vi "END SEM PROJECT ECG AND TEMP.vi"() -> ()   [LabVIEW 2014]
uses:
  <vilib>/MakerHub/LINX/Public/Peripherals/Analog/Analog Read 1 Chan.vi
  <vilib>/MakerHub/LINX/Public/Peripherals/Digital/Digital Write 1 Chan.vi
  <vilib>/MakerHub/LINX/Public/Peripherals/Analog/Analog Read N Chans.vi
  <vilib>/MakerHub/LINX/Public/Peripherals/Digital/Digital Write N Chans.vi
  <vilib>/MakerHub/LINX/Private/Local IO/LinxAnalogRead.vi
  <vilib>/MakerHub/LINX/Public/Utilities/Check Channel.vi
  <vilib>/MakerHub/LINX/Private/Local IO/LinxDigitalWrite.vi
  <vilib>/MakerHub/LINX/Public/Utilities/Open Serial.vi
  <vilib>/MakerHub/LINX/Private/Utilties/Generate Error.vi
  <vilib>/MakerHub/LINX/LMH-LINX.lvlib
panel:
  out "TEMPERATURE":dbl
  out "?":bool
  out "Thermometer":dbl(knob) scale=0.1..100.0
  in  "PORT":refnum<visa-resource-name>
  in  "?":bool
  out "PULSE":bool
  out "ECG":dbl(graph)
  # "ELECTROCARDIOGRAPH"
  # "BODY TEMPERATURE"
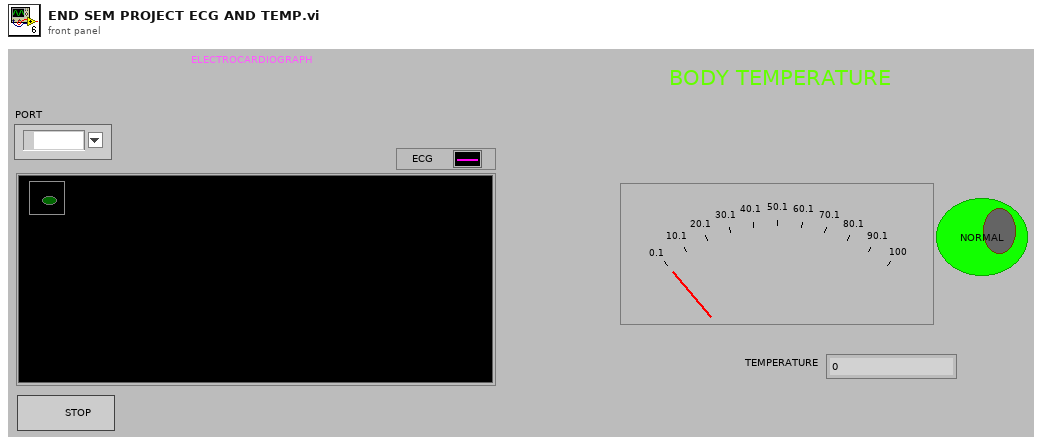
[diagram p1: front panel]
types:
  T1 = typedef "LMH-LINX.lvlib/LINX Ref.ctl" = cluster{"IO":T2, "Interface":T3, "LINX Device Config":T4}
  T2 = typedef "LMH-LINX.lvlib/Platform.ctl" = enum16{"Remote", "Local"}
  T3 = typedef "LMH-LINX.lvlib/Interface.ctl" = enum16{"Serial", "TCP"}
  T4 = typedef "LMH-LINX.lvlib/Device.lvlib/LINX Device Config.ctl" = cluster{"Interface":T3, "COM Port":refnum<visa-resource-name>, "TCP Configuration":T5, "Device Family":u8, "Device ID":u8, "Device Name":string, "TCP Ref":refnum<k5>, "Channels":T6}
  T5 = typedef "LMH-LINX.lvlib/Device.lvlib/TCP Config.ctl" = cluster{"IP Address":string, "Port":u16}
  T6 = typedef "LMH-LINX.lvlib/Channels.ctl" = cluster{"DI":u8[], "DO":u8[], "AI":u8[], "AO":u8[], "PWM":u8[], "QE":u8[], "UART":u8[], "I2C 2":u8[], "SPI":u8[], "CAN":u8[], "Servo":u8[], "AI Ref (V)":dbl, "AI Resolution (Bits)":u8, "AO Ref (V)":dbl, "AO Resolution (Bits)":u8}
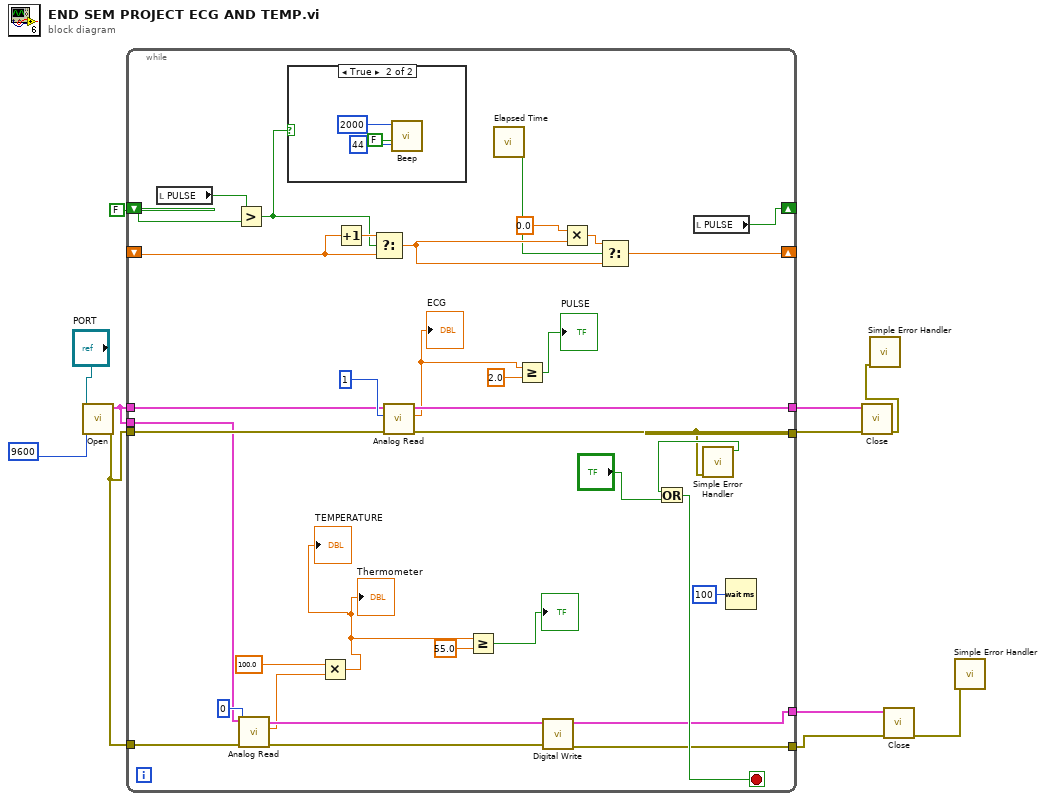
[diagram p0: block diagram]
diagram:
  n1 = call-poly <vilib>:"Open.vi"("Baud Rate Override"=9600 ("code"), "Serial Port"="PORT") -> ("Error Out"=w5:errorcluster, "LINX Resource"=w2:T1)  [unwired: 7 in, 1 out]
  n2 = while {
    tunnel: w5 -> [w46]
    tunnel: [w39] -> w11
    tunnel: w2 -> [w21]
    tunnel: [w43] -> w10
    shift-right: [w30] -> _
    shift-left: _ -> [w34]
    shift-right: [w29] -> _
    shift-left: FALSE -> [w33]
    tunnel: w5 -> [w13]
    tunnel: [w24] -> w4
    tunnel: [w23] -> w3
    tunnel: w2 -> [w12]
    stop <- w41 stop-if-true
    n3 = local read "PULSE"() -> (w32:bool)
    n4 = Greater?(x=w32, y=w33) -> (0:w28:bool)
    n5 = call-poly <vilib>:"Analog Read.vi"("Error In"=w13, "Analog Channel"=u8 0, "LINX Resource"=w12) -> ("Error Out"=w25:errorcluster, "Voltage"=w20:dbl, "LINX Resource"=w22:T1)  [unwired: 5 in, 1 out]
    n6 = case shown="True" w28 {
      frame False {
      }
      frame True {
        n7 = call <vilib>:"Beep.vi"("use system alert? (T)"=FALSE, "duration (msec)"=u32 44, "frequency (Hz)"=u32 2000) -> ()  [unwired: 9 in]
      }
    }
    n8 = Multiply(x=100.0, y=w20) -> (x*y=w17:dbl)
    "Thermometer" <- w17
    "TEMPERATURE" <- w17
    n9 = Increment(x=w34) -> (x+1=w35:dbl)
    n10 = Select(t=w35, s=w28, f=w34) -> (s? t:f=w37:dbl)
    n11 = call-poly <vilib>:"Analog Read.vi"("Error In"=w46, "Analog Channel"=1, "LINX Resource"=w21) -> ("Error Out"=w39:errorcluster, "Voltage"=w26:dbl, "LINX Resource"=w43:T1)  [unwired: 5 in, 1 out]
    "ECG" <- w26
    n12 = Greater Or Equal?(x=w17, y=55.0) -> (x >= y?=→"?":bool)
    n13 = call "Elapsed Time"() -> ("Time has Elapsed"=w31:bool)  [unwired: 12 in, 7 out]
    n14 = Greater Or Equal?(x=w26, y=2.0) -> (x >= y?=→"PULSE":bool)
    n15 = call-poly <vilib>:"Digital Write.vi"("Error In"=w25, "LINX Resource"=w22) -> ("Error Out"=w24:errorcluster, "LINX Resource"=w23:T1)  [unwired: 8 in]
    n16 = Multiply(x=0.0, y=w37) -> (x*y=w38:dbl)
    n17 = Select(t=w38, s=w31, f=w37) -> (s? t:f=w30:dbl)
    n18 = local read "PULSE"() -> (w29:bool)
    n19 = call <vilib>:"Simple Error Handler.vi"("error in (no error)"=w39) -> ("error?"=w40:bool)  [unwired: 4 in, 4 out]
    n20 = Or(x=w40, y="?") -> (x .or. y?=w41:bool)
    n21 = Wait (ms)(milliseconds to wait=u32 100) -> ()  [unwired: 1 out]
  }
  n22 = call <vilib>:"Close.vi"("Error In"=w11, "LINX Resource"=w10) -> ("Error Out"=w7:errorcluster)  [unwired: 9 in]
  n23 = call <vilib>:"Simple Error Handler.vi"("error in (no error)"=w7) -> ()  [unwired: 4 in, 5 out]
  n24 = call <vilib>:"Close.vi"("Error In"=w4, "LINX Resource"=w3) -> ("Error Out"=w1:errorcluster)  [unwired: 9 in]
  n25 = call <vilib>:"Simple Error Handler.vi"("error in (no error)"=w1) -> ()  [unwired: 4 in, 5 out]
